vi "AFMss_control_DelayObserver_trajTrack_extend.vi"() -> ()   [LabVIEW 2017]
uses:
  controls/controlParams_tracktraj.ctl
  controls/Xdelay.ctl
  <vilib>/rvi/Emulation/niFpgaGetClockAttributes.vi
  <vilib>/rvi/Emulation/niFpgaSctlEmulationGetInTimedLoop.vi
  <vilib>/rvi/Emulation/niFpgaEmulationReportErrorSimple.vi
  <vilib>/rvi/eio/common/nirviEmuTemplateMethod_errors.vi
  <vilib>/rvi/Emulation/niFpgaCriticalErrorInLSC.vi
  <vilib>/rvi/DataTransferAndStorage/Container/Common/niFpgaContainerExecOnDevCompGetState.vi
  <vilib>/rvi/Emulation/niFpgaEmulationIsFPGAContextNoSignature.vi
  <vilib>/rvi/DataTransferAndStorage/Container/Common/niFpgaContainerGetUniqueNameForEmu.vi
  <vilib>/rvi/Memory/Memory_Emulation/niFpgaMemoryEmulationCacheClearOnFirstRun.vi
  <vilib>/rvi/Memory/Memory_Emulation/nirvimemoryEmulationManagerCache_MakeExclusive.vi
  <vilib>/rvi/Memory/Memory_Emulation/niFpgaMemoryEmulationValidateCache.vi
  <vilib>/rvi/Memory/Memory_Emulation/nirvimemoryEmulationManagerCache_InsertValue.vi
  <vilib>/Utility/error.llb/Clear Errors.vi
  <vilib>/rvi/Memory/Memory_Emulation/nirvimemoryEmulationManagerCache_ReleaseExclusive.vi
  <vilib>/rvi/Memory/Memory_Emulation/nirvimemoryEmulationManagerCache_GetValue.vi
  <vilib>/rvi/Memory/Memory_Emulation/nirvimemoryEmulationManagerCache_SetValue.vi
  <vilib>/rvi/Emulation/niFpgaProcessEmulError.vi
  <vilib>/rvi/interface/RandomDataEmulation/niFpgaRandomDataHandleErrors.vi
  <vilib>/eio/EIONode/EIONode.xnode
  <vilib>/rvi/DataTransferAndStorage/Container/XNode/niFpgaContainer.xnode
  <vilib>/rvi/DataTransferAndStorage/Register/Emulation/niFpgaRegisterEmulationRefIn.vi
  <vilib>/rvi/interface/RandomDataEmulation/nirviRandomDataFpgaReadWriteTemplate.vi
  <vilib>/rvi/FXPMathLib/FxpSub/XNode/nifxpmath_Sub.xnode
  <vilib>/rvi/FXPMathLib/sim/FxpSim.dll
panel:
  in  "N":i32
  out "Xd_out(k+1)":T1
  out "yk":sgl
  out "u_xk":sgl
  out "yuxk TO":bool
  out "YK TO":bool
  out "UK TO":bool
  in  "Cluster":T2={"umax"=3.0, "y_ref(k)"=0.0, "Ki"=0.0, "y(k) (from plant)"=0.0, "ND"=0, "NS"=0, "u_Kx_ref(k)"=0.0} {"u_Kx_ref(k)" format="%#_13g"; "Ki" format="%#_13g"; "y_ref(k)" format="%#_13g"; "umax" format="%#_13g"}
  out "Unstable Traj":bool
  out "ND":i16=2
  out "Loop Done":bool
  in  "Settle Ticks":i16=1000
  in  "False  = cont run":bool=TRUE
  in  "Abort":bool=TRUE
  in  "iters":i16=1
  in  "ymax":sgl=4.0 format="%#_13g"
  in  "TsTicks":i16
  out "Loop Ticks (benchmark)":i16
  out "NS":i16=2
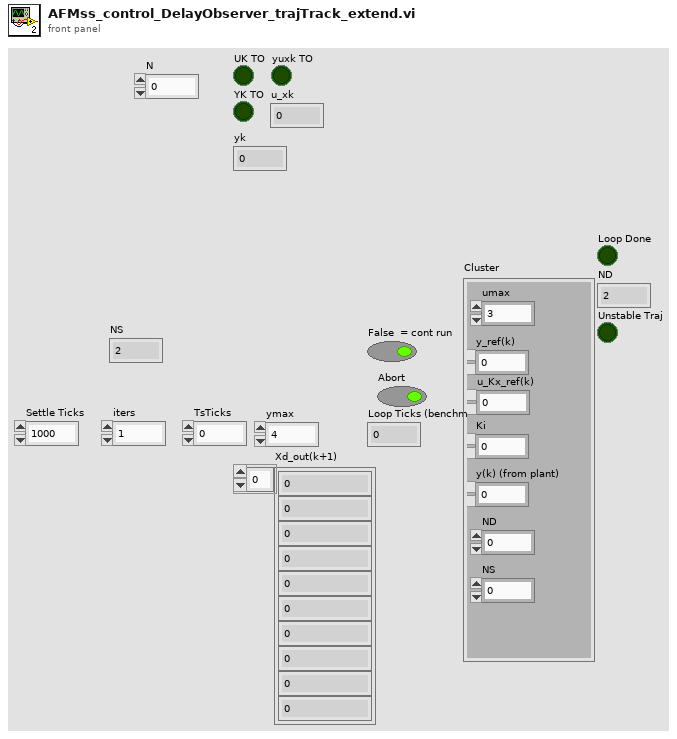
[diagram p1: front panel]
types:
  T1 = typedef "Xdelay.ctl" = sgl[]
  T2 = typedef "controlParams_tracktraj.ctl" = cluster{"umax":sgl, "y_ref(k)":sgl, "Ki":sgl, "y(k) (from plant)":sgl, "ND":i16, "NS":i16, "u_Kx_ref(k)":sgl}
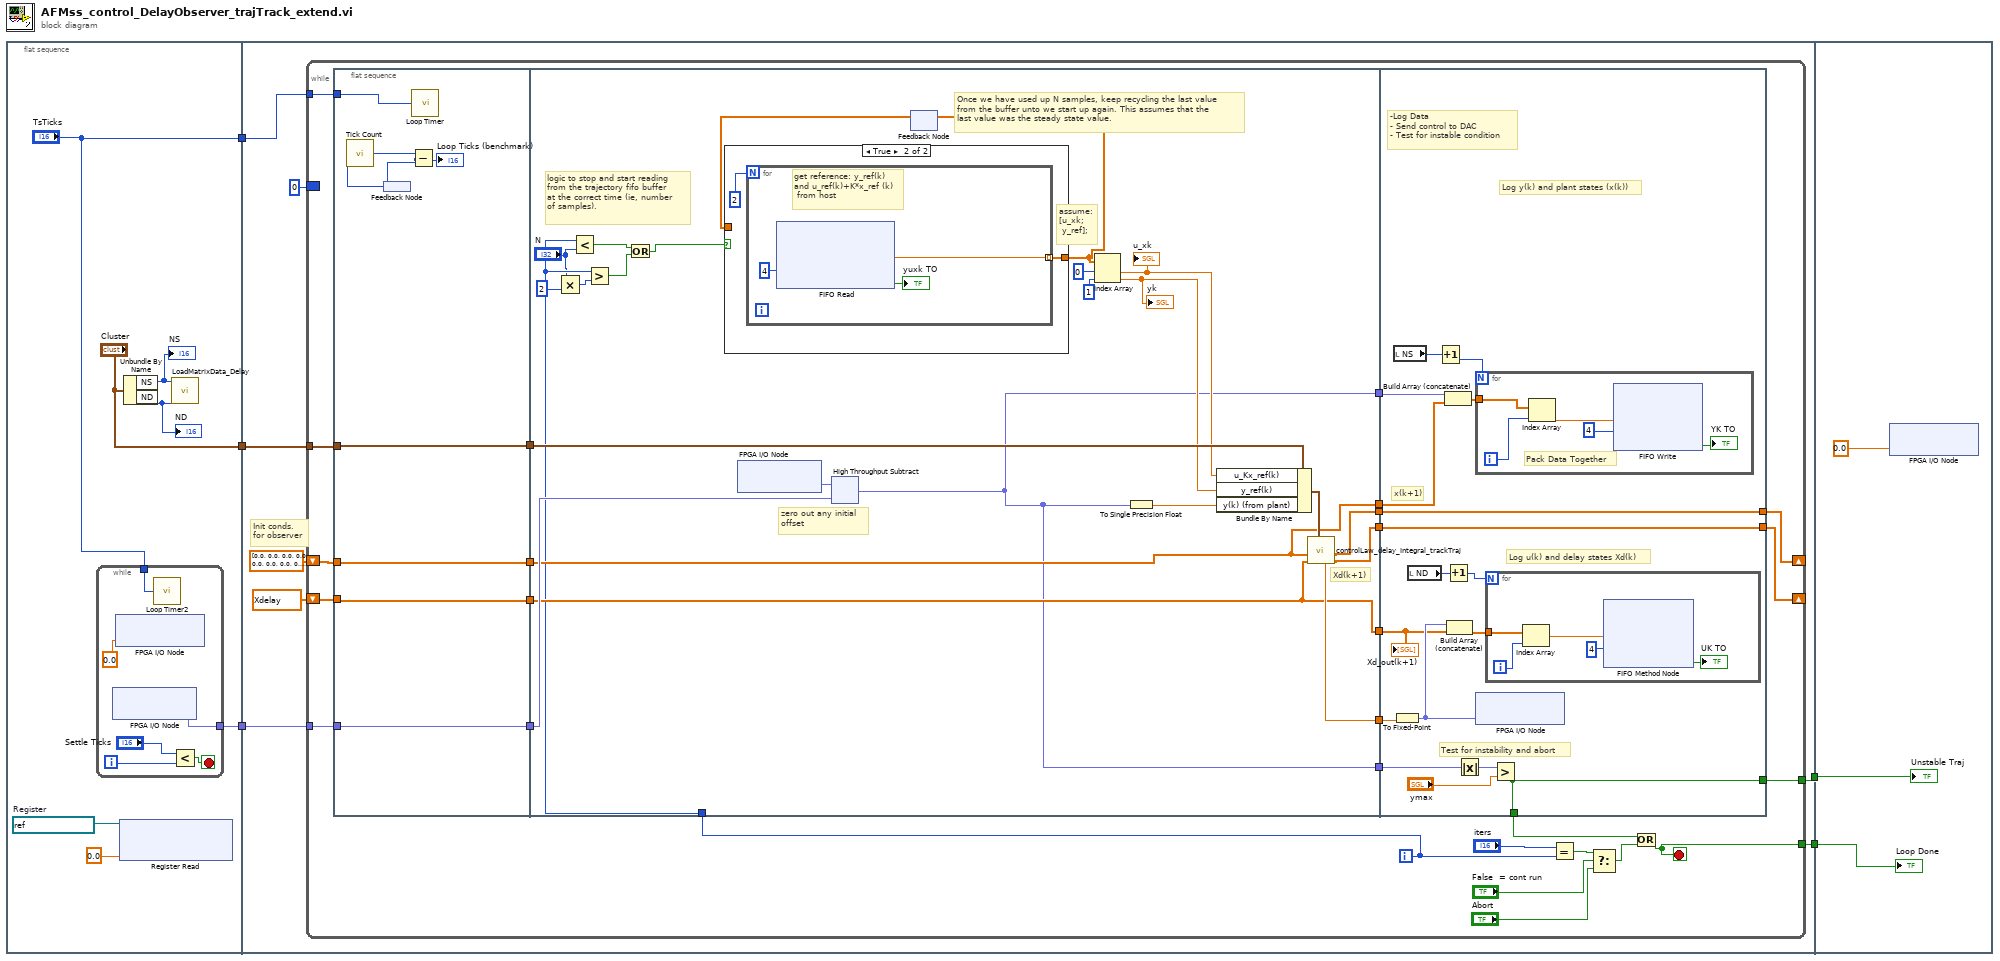
[diagram p0: block diagram]
diagram:
  n1 = flat-sequence {
    tunnel: ["TsTicks"] -> w5
    tunnel: [w12] -> w4
    tunnel: ["Cluster"] -> w2
    tunnel: w5 -> [w25]
    tunnel: w4 -> [w24]
    tunnel: [w21] -> w3
    tunnel: w2 -> [w20]
    tunnel: [w19] -> w1
    tunnel: w3 -> [w120]
    tunnel: w1 -> [w119]
    frame #0 {
      w10 = refnum<k21> "accumulator"  # Register
      # "Load Matrix Data"
      n2 = while {
        tunnel: [w18] -> w12
        tunnel: "TsTicks" -> [w17]
        i -> [w13]
        stop <- w15 stop-if-true
        n3 = xnode "FPGA I/O Node"() -> ("Mod2/AI0"=w18:fxp<+/-,24,5>)  [unwired: 1 in, 1 out]
        n4 = xnode "FPGA I/O Node"("Mod1/AO0"=sgl 0.0) -> ()  [unwired: 1 in, 1 out]
        n5 = call "Loop Timer2"("Count(Ticks)"=w17) -> ()  [unwired: 1 out]
        n6 = Less?(x="Settle Ticks", y=w13) -> (x < y?=w15:bool)
      }
      n7 = xnode ("Register Read")("Data"=sgl 0.0, "Register In"=w10) -> ()  [unwired: 1 out]
      n8 = Unbundle By Name("Cluster") -> ("NS"=w8:i16, "ND"=w7:i16)
      "NS" <- w8
      "ND" <- w7
      n9 = call "LoadMatrixData_Delay.vi"("Nd"=w7, "NS"=w8) -> ()  [unwired: 9 in, 1 out]
    }
    frame #1 {
      # "Init conds.\nfor observer"
      n10 = while {
        border: i16 0 -> [_]
        tunnel: w25 -> [w45]
        tunnel: w24 -> [w43]
        shift-right: [w37] -> _
        shift-left: T1 [0.0, 0.0, 0.0, 0.0, 0.0, 0.0, 0.0, 0.0, 0.0, 0.0, 0.0, 0.0] ("Xd_out(k+1)") -> [w36]
        shift-right: [w31] -> _
        shift-left: sgl[] [0.0, 0.0, 0.0, 0.0, 0.0, 0.0, 0.0, 0.0, 0.0, 0.0, 0.0, 0.0, 0.0, 0.0, 0.0, 0.0, 0.0, 0.0, 0.0, 0.0, 0.0, 0.0, 0.0, 0.0, 0.0] ("x^(k+1) = Ax + Bu + Lye") -> [w40]
        tunnel: [w35] -> w21
        tunnel: w20 -> [w33]
        tunnel: [w32] -> w19
        i -> [w27]
        stop <- w35 stop-if-true
        n11 = flat-sequence {
          tunnel: w45 -> [w58]
          tunnel: w43 -> [w57]
          tunnel: [w57] -> w42
          tunnel: [w55] -> w41
          tunnel: w40 -> [w56]
          tunnel: [w56] -> w39
          tunnel: w36 -> [w55]
          tunnel: [w54] -> w34
          tunnel: w33 -> [w54]
          tunnel: [w79] -> w53
          tunnel: [w80] -> w52
          tunnel: [w72] -> w44
          tunnel: w42 -> [w85]
          tunnel: w41 -> [w74]
          tunnel: w39 -> [w73]
          tunnel: [w78] -> w38
          tunnel: w34 -> [w82]
          tunnel: [w74] -> w30
          tunnel: [w73] -> w29
          tunnel: [w72] -> w28
          tunnel: w27 -> [w67]
          tunnel: w53 -> [w94]
          tunnel: w52 -> [w101]
          tunnel: [w96] -> w51
          tunnel: w44 -> [w105]
          tunnel: w38 -> [w100]
          tunnel: [w100] -> w37
          tunnel: [w96] -> w32
          tunnel: [w94] -> w31
          tunnel: w30 -> [w95]
          tunnel: w29 -> [w93]
          tunnel: w28 -> [w92]
          frame #0 {
            n12 = call "Tick Count"() -> ("Tick Count(Ticks)"=w59:u32)
            n13 = feedback #1() -> (w60:u32)
            n14 = feedback-in #1(w59) -> ()
            n15 = Subtract(x=w59, y=w60) -> (x-y=→"Loop Ticks (benchmark)":u32)
            n16 = call "Loop Timer"("Count(Ticks)"=w58) -> ()  [unwired: 1 out]
          }
          frame #1 {
            # "Once we have used up N samples, keep recycling the last value\nfrom the buffer unto we start up again. This assumes that the \nlast value was the steady state value."
            # "logic to stop and start reading\nfrom the trajectory fifo buffer\nat the correct time (ie, number \nof samples)."
            # "assume:\n[u_xk;\n y_ref];"
            # "Xd(k+1)"
            # "zero out any initial \noffset"
            n17 = Multiply(x="N", y=2) -> (x*y=w66:i32)
            n18 = Less?(x=w67, y="N") -> (x < y?=w70:bool)
            n19 = Greater?(x=w67, y=w66) -> (0:w68:bool)
            n20 = Or(x=w70, y=w68) -> (x .or. y?=w69:bool)
            n21 = xnode "FPGA I/O Node"() -> ("Mod2/AI0"=w84:fxp<+/-,24,5>)  [unwired: 1 in, 1 out]
            n22 = xnode "High Throughput Subtract"("x"=w84, "y"=w85) -> ("x-y"=w72:fxp<+/-,40,6>)
            n23 = feedback #2() -> (w62:sgl[])  [unwired: 1 in]
            n24 = case shown="True" w69 {
              tunnel: [w86 w87] -> w63
              tunnel: w62 -> [w86 _]
              frame False {
              }
              frame True {
                n25 = for {
                  N: i16 2 -> [_]
                  tunnel: [w90] -> w87 mode=indexing
                  # "get reference: y_ref(k)\nand u_ref(k)+K*x_ref (k)\n from host"
                  n26 = xnode ("FIFO Read")("Timeout"=i16 4) -> ("Element"=w90:sgl, "Timed Out?"=→"yuxk TO":bool)  [unwired: 1 in, 1 out]
                }
              }
            }
            n27 = feedback-in #2(w63) -> ()
            n28 = Index Array(array=w63, index #1=i16 0, index #2=i16 1) -> (element #1=w76:sgl, element #2=w75:sgl)
            "u_xk" <- w76
            "yk" <- w75
            n29 = To Single Precision Float(number=w72) -> (single precision float=w83:sgl)
            n30 = Bundle By Name(cluster=w82, "u_Kx_ref(k)"=w76, "y_ref(k)"=w75, "y(k) (from plant)"=w83) -> (w81:T2)
            n31 = call "controlLaw_delay_Integral_trackTraj.vi"("Cluster"=w81, "Xd_in"=w74, "x^(k)"=w73) -> ("Xd_out(k+1)"=w78:T1, "x^(k+1) = Ax + Bu + Lye"=w79:sgl[], "u(k) (saturated)"=w80:sgl)  [unwired: 6 in]
          }
          frame #2 {
            # "x(k+1)"
            # "Log u(k) and delay states Xd(k)"
            # "Log y(k) and plant states (x(k))"
            # "-Log Data\n- Send control to DAC\n- Test for instable condition"
            # "Test for instability and abort"
            n32 = local read "NS"() -> (w102:i16)
            n33 = To Fixed-Point(number=w101) -> (fixed-point=w97:fxp<+/-,32,6>)  [unwired: 1 in]
            n34 = local read "ND"() -> (w104:i16)
            n35 = Increment(x=w102) -> (x+1=w103:i16)
            n36 = Build Array (concatenate)(w105, w93) -> (w106:sgl[])
            n37 = Increment(x=w104) -> (x+1=w98:i16)
            n38 = Build Array (concatenate)(w97, w95) -> (w99:sgl[])
            n39 = Absolute Value(x=w92) -> (abs(x)=w108:fxp<+,40,6>)
            n40 = for {
              N: w103 -> [_]
              tunnel: w106 -> [w116]
              i -> [w117]
              # "Pack Data Together"
              n41 = Index Array(array=w116, index=w117) -> (element=w115:sgl)
              n42 = xnode ("FIFO Write")("Element"=w115, "Timeout"=i16 4) -> ("Timed Out?"=→"YK TO":bool)  [unwired: 1 in, 1 out]
            }
            n43 = xnode "FPGA I/O Node"("Mod1/AO0"=w97) -> ()  [unwired: 1 in, 1 out]
            n44 = for {
              N: w98 -> [_]
              tunnel: w99 -> [w110]
              i -> [w112]
              n45 = Index Array(array=w110, index=w112) -> (element=w111:sgl)
              n46 = xnode ("FIFO Method Node")("Element"=w111, "Timeout"=i16 4) -> ("Timed Out?"=→"UK TO":bool)  [unwired: 1 in, 1 out]
            }
            n47 = Greater?(x=w108, y="ymax") -> (0:w96:bool)
            "Xd_out(k+1)" <- w95
          }
        }
        n48 = Equal?(x="iters", y=w27) -> (x = y?=w48:bool)
        n49 = Select(t=w48, s="False  = cont run", f="Abort") -> (s? t:f=w49:bool)
        n50 = Or(x=w51, y=w49) -> (x .or. y?=w35:bool)
      }
    }
    frame #2 {
      n51 = xnode "FPGA I/O Node"("Mod1/AO0"=sgl 0.0) -> ()  [unwired: 1 in, 1 out]
      "Loop Done" <- w120
      "Unstable Traj" <- w119
    }
  }
